vi "UI_Loading_Unit.vi"() -> ()   [LabVIEW 2014]
panel:
  out "DATA":T1
  in  "退出":bool
  # "加载单元监测参数"
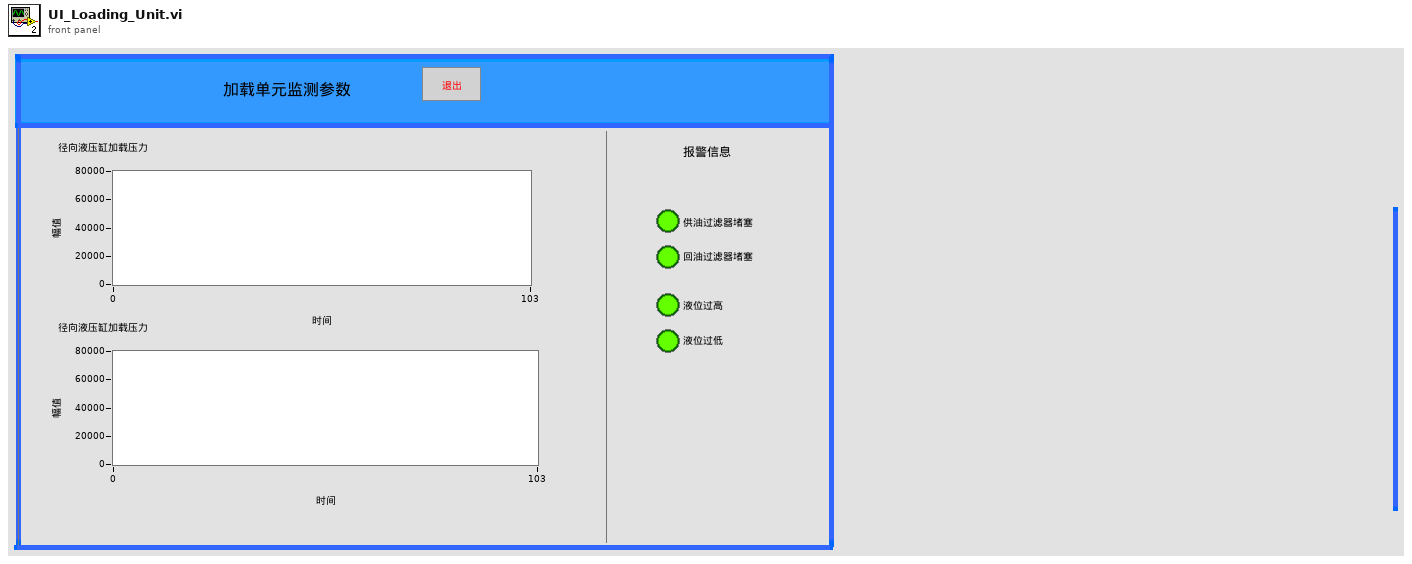
[diagram p1: front panel]
types:
  T1 = cluster{"径向液压缸加载压力":cluster{sgl, sgl, "径向油缸加载压力":u16}, "轴向液压缸加载压力":cluster{sgl, sgl, "轴向油缸加载压力":u16}, "报警信息":cluster{"加载单元供油过滤器堵塞":bool, "加载单元回油过滤器堵塞":bool, "加载单元液位过高":bool, "加载单元单元液位过低":bool}}
  T2 = cluster{"径向油缸加载压力":u16, "轴向油缸加载压力":u16, "油箱1油液温度":u16, "润滑油温度":u16, "油箱2油液温度":u16, "试验轴承供油压力":u16, "试验轴承供油流量":u16, "陪试轴承供油流量":u16, "陪试轴承供油压力":u16, "陪试轴承供油温度":u16, "液压子系统状态字":cluster{"加载单元":cluster{"供油过滤器堵塞报警":bool, "回油过滤器堵塞报警":bool, "液位过高报警":bool, "液位过低报警":bool}, "试验轴承单元":cluster{"加热装置异常报警":bool, "油箱1液位过高报警":bool, "油箱1液位过低报警":bool, "油箱2液位过高报警":bool, "油箱2液位过低报警":bool, "供油过滤器堵塞报警":bool, "循环回路过滤器堵塞报警":bool, "回油过滤器堵塞报警":bool}, "陪试轴承单元":cluster{"供油过滤器1堵塞报警":bool, "供油过滤器2堵塞报警":bool, "回油过滤器堵塞报警":bool, "油箱液位过高报警":bool, "油箱液位过低报警":bool}}}
  T3 = cluster{"供油过滤器堵塞报警":bool, "回油过滤器堵塞报警":bool, "液位过高报警":bool, "液位过低报警":bool}
  T4 = cluster{cluster{sgl, sgl, "径向油缸加载压力":u16}, cluster{sgl, sgl, "轴向油缸加载压力":u16}, "加载单元":cluster{"供油过滤器堵塞报警":bool, "回油过滤器堵塞报警":bool, "液位过高报警":bool, "液位过低报警":bool}}
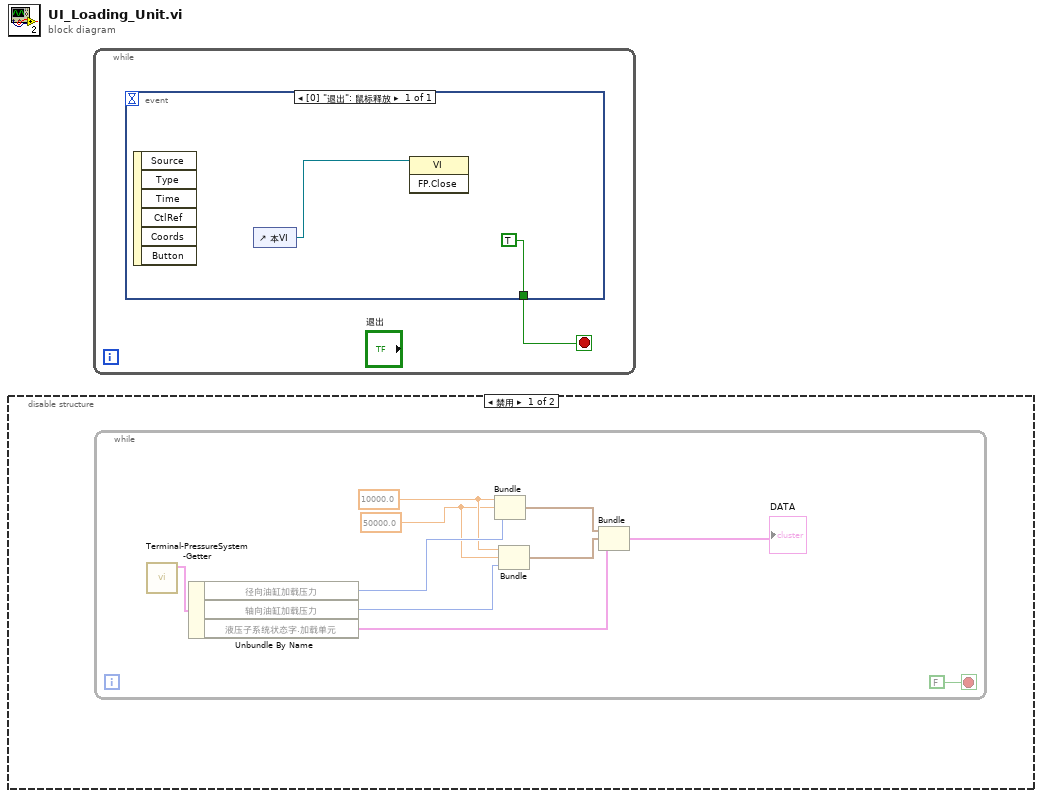
[diagram p0: block diagram]
diagram:
  n1 = disable-structure shown="禁用" {
    frame Disabled {
      n2 = while {
        stop <- FALSE stop-if-true
        w7 = sgl 50000.0
        w8 = sgl 10000.0
        n3 = call "Terminal-PressureSystem-Getter.vi"() -> ("设备信息"=w10:T2)  [unwired: 10 in, 1 out]
        n4 = Unbundle By Name(w10) -> ("径向油缸加载压力"=w9:u16, "轴向油缸加载压力"=w6:u16, "液压子系统状态字.加载单元"=w3:T3)
        n5 = Bundle(w8, w7, "径向油缸加载压力"=w9) -> (w5:cluster{sgl, sgl, "径向油缸加载压力":u16})  [unwired: 1 in]
        n6 = Bundle(w8, w7, "轴向油缸加载压力"=w6) -> (w4:cluster{sgl, sgl, "轴向油缸加载压力":u16})  [unwired: 1 in]
        n7 = Bundle(w5, w4, "加载单元"=w3) -> (→"DATA":T4)  [unwired: 1 in]
      }
    }
    frame Enabled {
    }
  }
  n8 = while {
    stop <- w11 stop-if-true
    n9 = event shown="[0] \"退出\": 鼠标释放" {
      selector: _ -> [_]
      dyn-events: _ -> [_]
      timeout: _ -> [_]
      tunnel: [TRUE] -> w11
      event "退出": Mouse Up {
        n10 = event-data() -> ()  [unwired: 1 in, 6 out]
        n11 = control-ref of="本VI"() -> (w13:refnum<vi>)
        n12 = invoke class="VI" method="FP.Close"(reference=w13) -> ()  [unwired: 2 in, 3 out]
      }
    }
  }
